vi "Initialize Local Variable.vi"(8 "error in":errorcluster, 11 "Timed Node in":refnum<class "AMS Power Supply Template.lvclass">) -> (0 "error out":errorcluster, 1 "Main to gRPC":T1, 2 "gRPC to Main":T2, 3 "Timed Node out":refnum<class "AMS Power Supply Template.lvclass">)   [LabVIEW 2023, in "AMS Power Supply Template.lvlib" / "AMS Power Supply Template.lvclass"]
uses:
  AMS Power Supply Template.lvclass
  Type Defs/gRPC to Main.ctl
  Type Defs/Main to gRPC.ctl
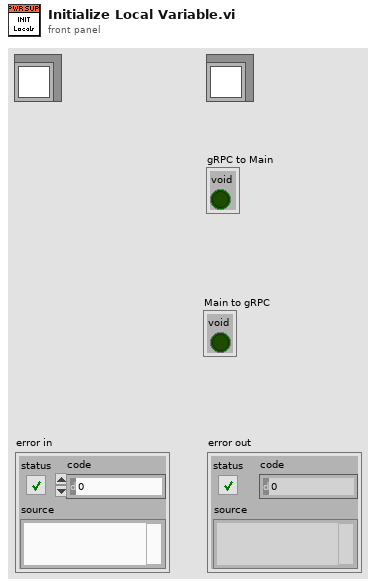
[diagram p1: front panel]
types:
  T1 = typedef "AMS Power Supply Template.lvlib/AMS Power Supply Template.lvclass/Main to gRPC.ctl" = cluster{"void":bool}
  T2 = typedef "AMS Power Supply Template.lvlib/AMS Power Supply Template.lvclass/gRPC to Main.ctl" = cluster{"void":bool}
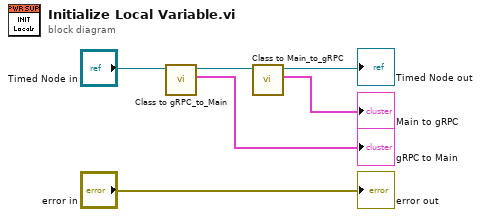
[diagram p0: block diagram]
diagram:
  n1 = call "Class to gRPC_to_Main.vi"("Timed Node in"="Timed Node in") -> ("gRPC to Main"=→"gRPC to Main":T2, "Timed Node out"=w5:refnum<class "AMS Power Supply Template.lvclass">)  [unwired: 9 in]
  n2 = call "Class to Main_to_gRPC.vi"("Timed Node in"=w5) -> ("Main to gRPC"=→"Main to gRPC":T1, "Timed Node out"=→"Timed Node out":refnum<class "AMS Power Supply Template.lvclass">)  [unwired: 9 in]
  "error out" <- "error in"
